vi "CCON To Byte.vi"(11 "CCON":T1) -> (3 "Numeric":u8)   [LabVIEW 2022 SP3, in "FHPP.lvclass"]
uses:
  FHPP.lvclass
  FHPP.lvclass/FHPP.ctl
  TypeDefs/CCON.ctl
  TypeDefs/Operating Mode.ctl
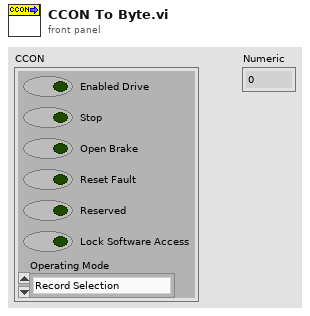
[diagram p1: front panel]
types:
  T1 = typedef "FHPP.lvclass/CCON.ctl" = cluster{"Enabled Drive":bool, "Stop":bool, "Open Brake":bool, "Reset Fault":bool, "Reserved":bool, "Lock Software Access":bool, "Operating Mode":T2}
  T2 = typedef "FHPP.lvclass/Operating Mode.ctl" = enum16{"Record Selection", "Direct Mode", "Reserved 1", "Reserved 2"}
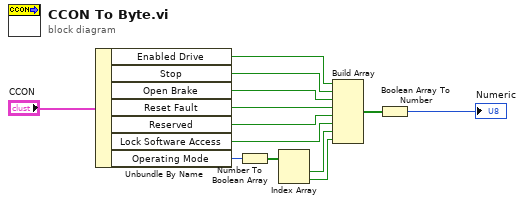
[diagram p0: block diagram]
diagram:
  n1 = Unbundle By Name("CCON") -> ("Enabled Drive"=w2:bool, "Stop"=w3:bool, "Open Brake"=w4:bool, "Reset Fault"=w5:bool, "Reserved"=w6:bool, "Lock Software Access"=w7:bool, "Operating Mode"=w8:T2)
  n2 = Number To Boolean Array(number=w8) -> (Boolean array=w9:bool[])
  n3 = Index Array(array=w9) -> (element #1=w10:bool, element #2=w11:bool)  [unwired: 2 in]
  n4 = Build Array(w2, w3, w4, w5, w6, w7, w10, w11) -> (w12:bool[])
  n5 = Boolean Array To Number(Boolean array=w12) -> (number=→"Numeric":u8)
